vi "FPGA Compile Steps.vi"   [LabVIEW 2012]
uses:
  Type Defs/WSVCAP SHL Function Enum.ctl
  Type Defs/WSVCAP SHL Top Level Control Operation Enum.ctl
  Type Defs/WSVCAP SHL I2C FPGA Enum.ctl
  Type Defs/WSVCAP SHL FPGA VI Reference.ctl
  Type Defs/WSVCAP SHL FPGA Interface Instance Ref Cluster.ctl
  Type Defs/WSVCAP SHL Manage FPGA Top Level Controls VI Ref.ctl
panel:
  # "See Block Diagram for Step by Step Instructions for AFTER you have created a new bitfile"
types:
  T1 = typedef "WSVCAP SHL I2C FPGA Enum.ctl" = enum16{"RIO0", "RIO1"}
  T2 = typedef "WSVCAP SHL Top Level Control Operation Enum.ctl" = enum16{"Initialize", "Set Control", "Read Control", "Close"}
  T3 = typedef "WSVCAP SHL Function Enum.ctl" = enum16{"Initialize", "Configure I2C", "Configure RFFE", "Write I2C", "Read I2C", "Write RFFE", "Read RFFE", "Start RFFE Cycle", "Stop RFFE Cycle", "Get Status", "Close"}
  T4 = typedef "WSVCAP SHL Manage FPGA Top Level Controls VI Ref.ctl" = refnum<vi>
  T5 = typedef "WSVCAP SHL FPGA Interface Instance Ref Cluster.ctl" = cluster{"Core Instance ID":refnum<vi>, "ST MGR Instance ID":refnum<vi>}
  T6 = typedef "WSVCAP SHL FPGA VI Reference.ctl" = refnum<k20>
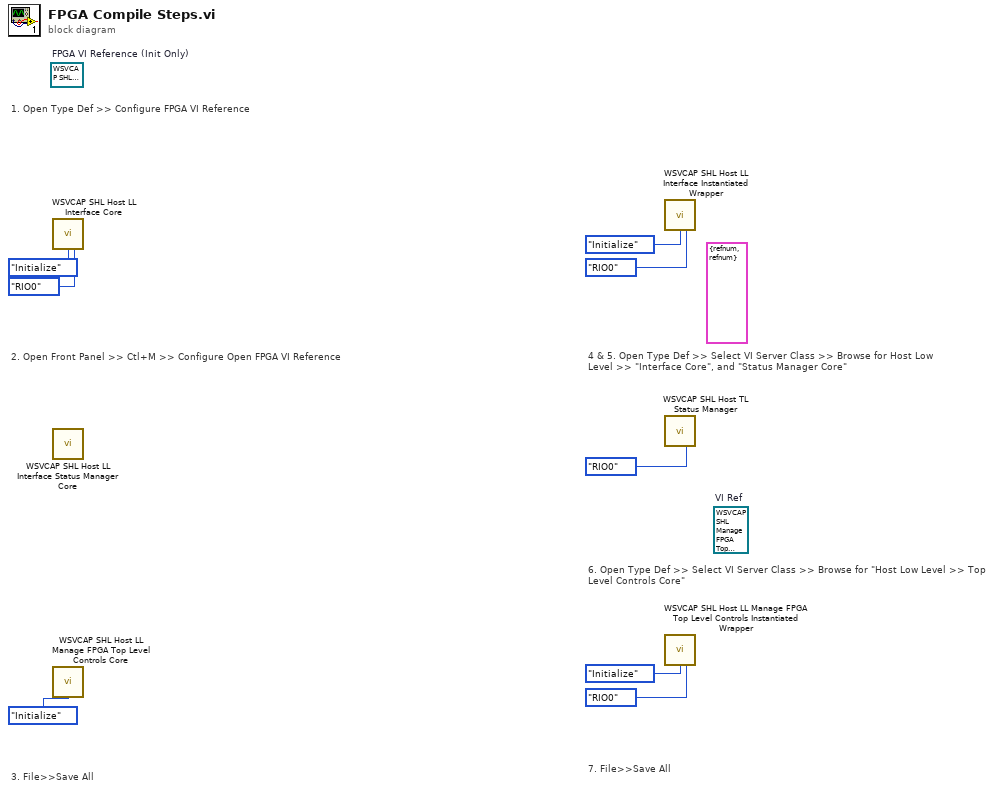
[diagram p0: block diagram]
diagram:
  (unwired) T4 refnum  # VI Ref
  (unwired) T5 {"Core Instance ID"=refnum, "ST MGR Instance ID"=refnum} ("Instance IDs")
  (unwired) T6 refnum  # FPGA VI Reference (Init Only)
  # "7. File>>Save All"
  # "3. File>>Save All"
  # "6. Open Type Def >> Select VI Server Class >> Browse for \"Host Low Level >> Top Level Controls Core\""
  # "4 & 5. Open Type Def >> Select VI Server Class >> Browse for Host Low Level >> \"Interface Core\", and \"Status Manager Core\""
  # "1. Open Type Def >> Configure FPGA VI Reference"
  # "2. Open Front Panel >> Ctl+M >> Configure Open FPGA VI Reference"
  n1 = call "WSVCAP SHL Host LL Interface Core.vi"("Function"=WSVCAP_SHL_Function_Enum."Initialize", "FPGA"=WSVCAP_SHL_I2C_FPGA_Enum."RIO0") -> ()  [unwired: 11 in, 3 out]
  n2 = call "WSVCAP SHL Host LL Interface Status Manager Core.vi"() -> ()  [unwired: 14 in, 2 out]
  n3 = call "WSVCAP SHL Host LL Manage FPGA Top Level Controls Core.vi"("Operation"=WSVCAP_SHL_Top_Level_Control_Operation_Enum."Initialize") -> ()  [unwired: 13 in, 2 out]
  n4 = call "WSVCAP SHL Host LL Interface Instantiated Wrapper.vi"("Function"=WSVCAP_SHL_Function_Enum."Initialize", "FPGA"=WSVCAP_SHL_I2C_FPGA_Enum."RIO0") -> ()  [unwired: 11 in, 3 out]
  n5 = call "WSVCAP SHL Host TL Status Manager.vi"("FPGA"=WSVCAP_SHL_I2C_FPGA_Enum."RIO0") -> ()  [unwired: 13 in, 2 out]
  n6 = call "WSVCAP SHL Host LL Manage FPGA Top Level Controls Instantiated Wrapper.vi"("Operation"=WSVCAP_SHL_Top_Level_Control_Operation_Enum."Initialize", "FPGA"=WSVCAP_SHL_I2C_FPGA_Enum."RIO0") -> ()  [unwired: 12 in, 2 out]
